vi "Get_Thorlabs_Device_List.vi"(8 "error in (no error)":errorcluster) -> (0 "error out":errorcluster, 3 "Device List":string[][](array[string]))   [LabVIEW 2023]
uses:
  C:/Users/quantum/Documents/LVDAQ/UIs/TranslationStage_UI/Thorlabs.MotionControl.DeviceManagerCLI.dll
  Thorlabs.MotionControl.DeviceManagerCLI.dll
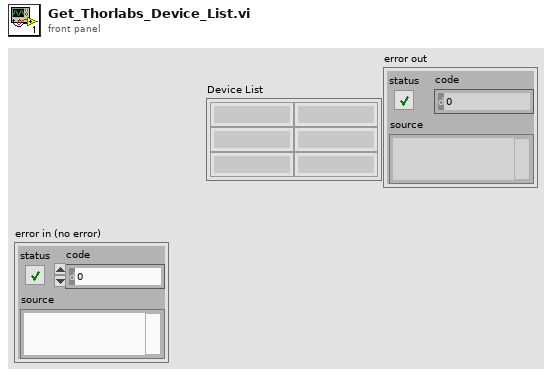
[diagram p1: front panel]
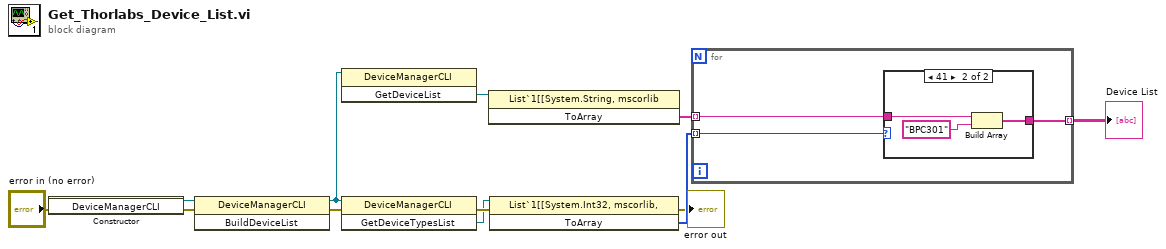
[diagram p0: block diagram]
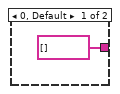
[diagram p2: hidden frame]
diagram:
  n1 = constructor class="DeviceManagerCLI"(error in="error in (no error)") -> (reference out=w2:refnum<k24>, error out=w3:errorcluster)  [unwired: 2 in, 1 out]
  n2 = invoke class="DeviceManagerCLI" method="BuildDeviceList"(reference=w2, error in=w3) -> (reference out=w7:refnum<k24>, error out=w6:errorcluster)  [unwired: 1 in, 1 out]
  n3 = invoke class="DeviceManagerCLI" method="GetDeviceList"(reference=w7) -> ("GetDeviceList"=w5:refnum<k24>)  [unwired: 2 in, 2 out]
  n4 = invoke class="DeviceManagerCLI" method="GetDeviceTypesList"(reference=w7, error in=w6) -> (error out=w9:errorcluster, "GetDeviceTypesList"=w8:refnum<k24>)  [unwired: 1 in, 1 out]
  n5 = invoke class="List`1[[System.String, mscorlib" method="ToArray"(reference=w5) -> ("ToArray"=w11:string[])  [unwired: 2 in, 2 out]
  n6 = invoke class="List`1[[System.Int32, mscorlib," method="ToArray"(reference=w8, error in=w9) -> (error out=→"error out":errorcluster, "ToArray"=w10:i32[])  [unwired: 1 in, 1 out]
  n7 = for {
    tunnel: w10 -> [w15] mode=indexing
    tunnel: w11 -> [w14] mode=indexing
    tunnel: [w13] -> w12 mode=indexing
    n8 = case shown="41" w15 {
      tunnel: w14 -> [_ w19]
      tunnel: [string[] [] w18] -> w13
      frame 0, Default {
      }
      frame 41 {
        n9 = Build Array(w19, "BPC301" ("element")) -> (w18:string[])
      }
    }
  }
  "Device List" <- w12
